vi "1A ReadFromFIFOPort3.vi"(10 "stop":bool) -> (2 "This is what I told you!":string)   [LabVIEW 2011]
doc: "Elizabeth Mahon\nBased off of example from LabView and IGVC 3.2.1 Read VectorNav.\nReads data from compass sensor on port 1 of the serial module from a FIFO and outputs it as a string.\nStarts as waiting, then when it reads $ (first element of compass string) starts reading and adds everything it reads together until it reaches *ss (where ss can be anything, the \"two digit checksum\"), and then stops and outputs the string.\nOnly reads the string once - must be run in a while loop for multiple readings.\nJust shuts down if it has an error. In the future, we might want to output if it has an error."
uses:
  <vilib>/rvi/interface/nirviOpenFPGA/nirviOpenFPGA.xnode
  <vilib>/rvi/interface/nirviMethod/nirviMethod.xnode
  <vilib>/FPGAPlugInAG/Dynamic/niLvFpga_ReadFifo_Dynamic.vi
  <vilib>/rvi/errors/niLvFpgaMergeErrorWithErrorCode.vi
  <vilib>/rvi/interface/nirviCloseFPGA/nirviCloseFPGA.xnode
  FPGA Bitfiles/SailBot_FPGATarget_WriteToFIFOPort3_7F5D412A.lvbitx
  1A-FPGA/1A Code/WriteToFIFOPort3.vi
  <vilib>/FPGAPlugInAG/Dynamic/niLvFpga_Close_Dynamic.vi
panel:
  out "Current Status":enum16{"Waiting", "Reading", "Time Out!"}(ring)
  out "Data":i16[](array[numeric])
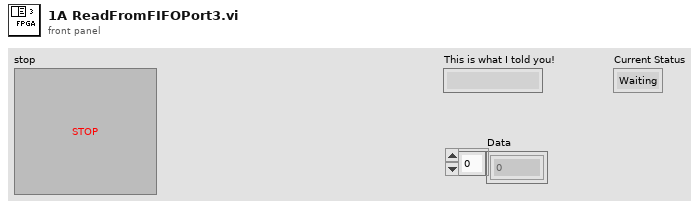
[diagram p1: front panel]
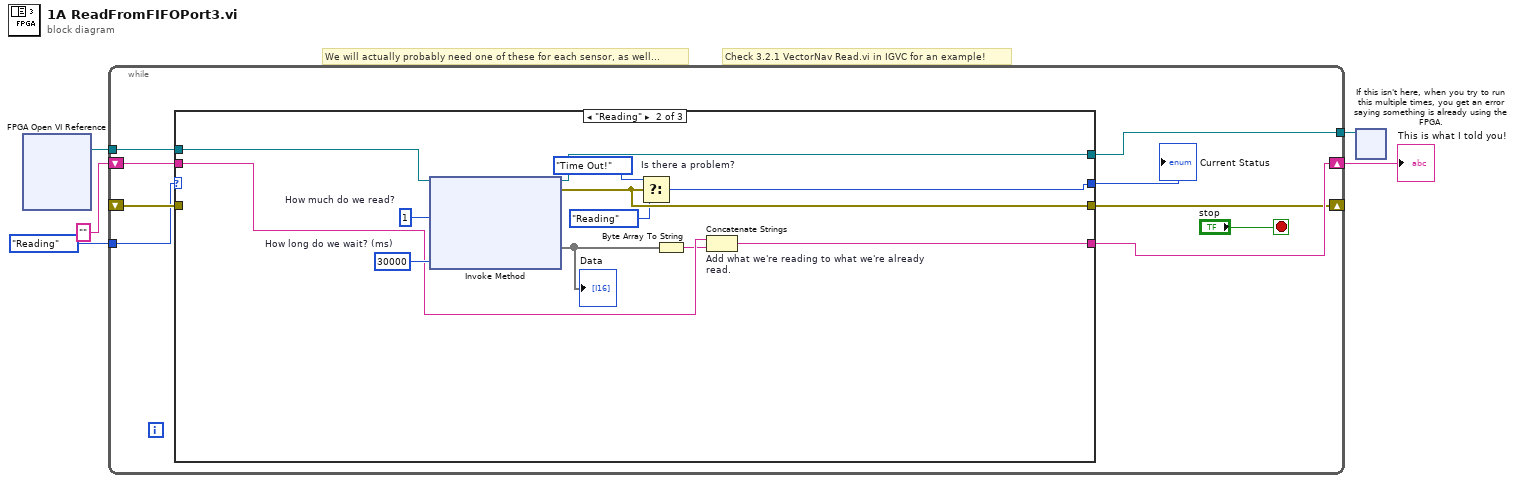
[diagram p0: block diagram]
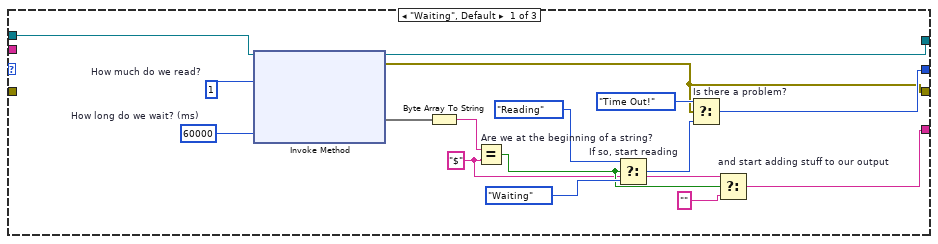
[diagram p2: hidden frame]
diagram:
  # "Check 3.2.1 VectorNav Read.vi in IGVC for an example!"
  # "We will actually probably need one of these for each sensor, as well..."
  n1 = xnode "FPGA Open VI Reference"() -> ("FPGA VI Reference Out"=w5:refnum<k20>)  [unwired: 2 in, 1 out]
  n2 = while {
    tunnel: w5 -> [w14]
    shift-right: [w12] -> w4
    shift-left: "" -> [w13]
    shift-right: [w11] -> _
    shift-left: _ -> [w10]
    tunnel: [w9] -> w2
    tunnel: enum16{"Waiting", "Reading", "Time Out!"}."Reading" ("Status") -> [w7]
    stop <- "stop" stop-if-true
    n3 = case shown="\"Reading\"" w7 {
      selector: w7 -> [_ _ w46]
      tunnel: w14 -> [w30 w40 w43]
      tunnel: w13 -> [_ w35 w45]
      tunnel: [w17 w36 w45] -> w12
      tunnel: [w21 w38 w46] -> w8
      tunnel: [w20 w37 w44] -> w11
      tunnel: w10 -> [_ _ w44]
      tunnel: [w29 w33 w43] -> w9
      frame "Waiting", Default {
        w16 = "$" ("x")
        w27 = 60000  # How long do we wait? (ms)
        w28 = u32 1  # How much do we read?
        n4 = xnode "Invoke Method"("FPGA VI Reference In"=w30, "Number of Elements"=w28, "Timeout (ms)"=w27) -> ("FPGA VI Reference Out"=w29:refnum<k20>, "error out"=w20:errorcluster, "Data"=w26:void[])  [unwired: 1 in, 1 out]
        n5 = Byte Array To String(unsigned byte array=w26) -> (string=w15:string)
        n6 = Equal? "Are we at the beginning of a string?"(x=w15, y=w16) -> (x = y?=w18:bool)
        n7 = Select "If so, start reading"(t=enum16{"Waiting", "Reading", "Time Out!"}."Reading", s=w18, f=enum16{"Waiting", "Reading", "Time Out!"}."Waiting" ("Current Status")) -> (s? t:f=w23:enum16{"Waiting", "Reading", "Time Out!"})
        n8 = Select "Is there a problem?"(t=enum16{"Waiting", "Reading", "Time Out!"}."Time Out!", s=w20, f=w23) -> (s? t:f=w21:enum16{"Waiting", "Reading", "Time Out!"})
        n9 = Select "and start adding stuff to our output"(t=w16, s=w18, f="") -> (s? t:f=w17:string)
      }
      frame "Reading" {
        w41 = 30000  # How long do we wait? (ms)
        w42 = u32 1  # How much do we read?
        n10 = xnode "Invoke Method"("FPGA VI Reference In"=w40, "Number of Elements"=w42, "Timeout (ms)"=w41) -> ("FPGA VI Reference Out"=w33:refnum<k20>, "error out"=w37:errorcluster, "Data"=w39:void[])  [unwired: 1 in, 1 out]
        "Data" <- w39
        n11 = Select "Is there a problem?"(t=enum16{"Waiting", "Reading", "Time Out!"}."Time Out!", s=w37, f=enum16{"Waiting", "Reading", "Time Out!"}."Reading" ("Status")) -> (s? t:f=w38:enum16{"Waiting", "Reading", "Time Out!"})
        n12 = Byte Array To String(unsigned byte array=w39) -> (string=w34:string)
        n13 = Concatenate Strings "Add what we're reading to what we're already read."(w35, w34) -> (w36:string)
      }
      frame "Time Out!" {
        # "error or something. Not sure what to do."
      }
    }
    "Current Status" <- w8
  }
  "This is what I told you!" <- w4
  n14 = xnode "If this isn't here, when you try to run\nthis multiple times, you get an error\nsaying something is already using the\nFPGA."("FPGA VI Reference In"=w2) -> ()  [unwired: 1 in, 1 out]
